vi "Draw FullyCustom Picture.vi"(5 "CycleAngle?":T1=TRUE caption="FPGA Simulation Angle Reference", 8 "error in (no error)":errorcluster, 11 "Tooth Angles":cluster{"Falling Edge":dbl, "Rising Edge":dbl}[](array[cluster])) -> (0 "error out":errorcluster, 3 "N Teeth M Missing View":picture)   [LabVIEW 2011, in "Engine Sim System Explorer.lvlib"]
uses:
  Engine Sim System Explorer.lvlib
  TypeDefs/AngleReference.ctl
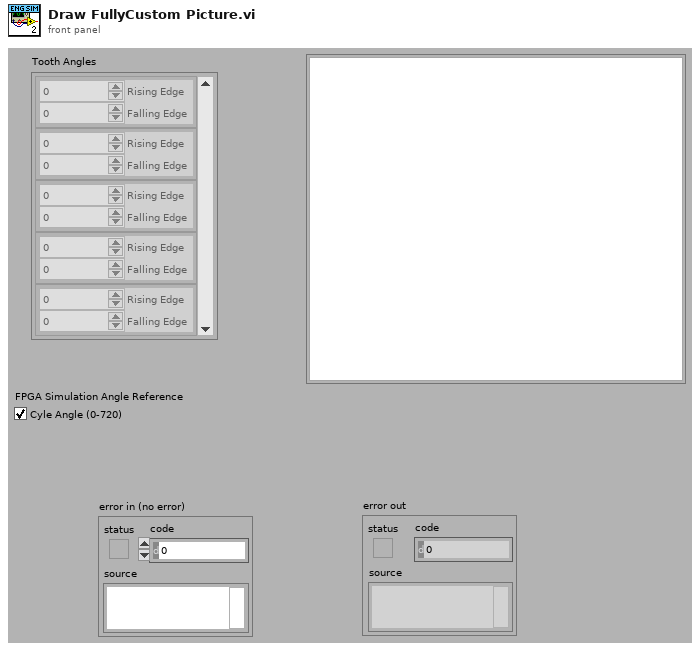
[diagram p1: front panel]
types:
  T1 = typedef "Engine Sim System Explorer.lvlib/AngleReference.ctl" = bool
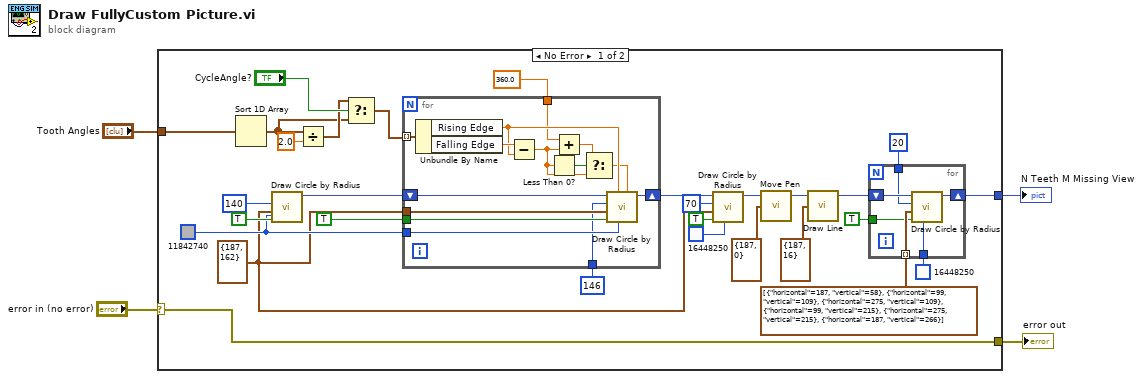
[diagram p0: block diagram]
diagram:
  n1 = case shown="No Error" "error in (no error)" {
    selector: "error in (no error)" -> [w12 w54]
    tunnel: [w15 _] -> w4
    tunnel: [w12 w54] -> w2
    tunnel: "Tooth Angles" -> [w11 _]
    frame No Error {
      w29 = u32 11842740 ("color(black)")
      w14 = cluster{"horizontal":i16, "vertical":i16} {"horizontal"=187, "vertical"=162} ("pixel center")
      n2 = Sort 1D Array(array=w11) -> (sorted array=w5:cluster{"Falling Edge":dbl, "Rising Edge":dbl}[])
      n3 = call <vilib>:"Draw Circle by Radius.vi"("color(black)"=w29, "fill?(F)"=TRUE, "pixel center"=w14, "radius"=i16 140) -> ("new picture"=w32:picture)  [unwired: 7 in]
      n4 = Divide(x=w5, y=2.0) -> (x/y=w7:cluster{"Falling Edge":dbl, "Rising Edge":dbl}[])
      n5 = Select(t=w7, s="CycleAngle?", f=w5) -> (s? t:f=w6:cluster{"Falling Edge":dbl, "Rising Edge":dbl}[])
      n6 = for {
        tunnel: TRUE ("fill?(F)") -> [w51]
        tunnel: w14 -> [w50]
        shift-right: [w52] -> w28
        shift-left: w32 -> [w53]
        tunnel: w29 -> [w49]
        tunnel: i16 146 ("radius") -> [w48]
        tunnel: w6 -> [w47] mode=indexing
        tunnel: 360.0 -> [w40]
        n7 = Unbundle By Name(w47) -> ("Rising Edge"=w45:dbl, "Falling Edge"=w46:dbl)
        n8 = Subtract(x=w46, y=w45) -> (x-y=w43:dbl)
        n9 = Less Than 0?(x=w43) -> (x < 0?=w44:bool)
        n10 = Add(x=w40, y=w43) -> (x+y=w42:dbl)
        n11 = Select(t=w42, s=w44, f=w43) -> (s? t:f=w41:dbl)
        n12 = call <vilib>:"Draw Circle by Radius.vi"("arc size(360)"=w41, "color(black)"=w49, "start angle(0)"=w45, "fill?(F)"=w51, "pixel center"=w50, "radius"=w48, "picture"=w53) -> ("new picture"=w52:picture)  [unwired: 4 in]
      }
      n13 = call <vilib>:"Draw Circle by Radius.vi"("color(black)"=u32 16448250, "fill?(F)"=TRUE, "pixel center"=w14, "radius"=i16 70, "picture"=w28) -> ("new picture"=w27:picture)  [unwired: 6 in]
      n14 = call <vilib>:"Move Pen.vi"("new position"=cluster{"x":i16, "y":i16} {"x"=187, "y"=0} ("end point"), "picture"=w27) -> ("new picture"=w22:picture)  [unwired: 3 in]
      n15 = call <vilib>:"Draw Line.vi"("picture"=w22, "end point"=cluster{"x":i16, "y":i16} {"x"=187, "y"=16}) -> ("new picture"=w20:picture)  [unwired: 7 in]
      n16 = for {
        shift-right: [w38] -> w15
        shift-left: w20 -> [w39]
        tunnel: i16 20 ("radius") -> [w37]
        tunnel: cluster{"horizontal":i16, "vertical":i16}[] [{"horizontal"=187, "vertical"=58}, {"horizontal"=99, "vertical"=109}, {"horizontal"=275, "vertical"=109}, {"horizontal"=99, "vertical"=215}, {"horizontal"=275, "vertical"=215}, {"horizontal"=187, "vertical"=266}] -> [w36] mode=indexing
        tunnel: TRUE ("fill?(F)") -> [w35]
        tunnel: u32 16448250 ("color(black)") -> [w34]
        n17 = call <vilib>:"Draw Circle by Radius.vi"("color(black)"=w34, "fill?(F)"=w35, "pixel center"=w36, "radius"=w37, "picture"=w39) -> ("new picture"=w38:picture)  [unwired: 6 in]
      }
    }
    frame Error {
    }
  }
  "N Teeth M Missing View" <- w4
  "error out" <- w2
